vi "End Drag.vi"(8 "error in (no error)":errorcluster, 11 "FSM in":refnum<class "FSM.Node.lvclass">) -> (0 "error out":errorcluster, 3 "FSM out":refnum<class "FSM.Node.lvclass">)   [LabVIEW 2015, in "FSM.Node.lvclass"]
uses:
  FSM.Node.lvclass
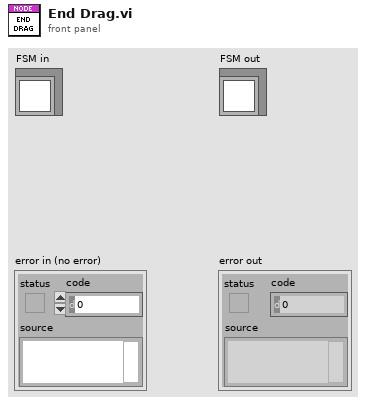
[diagram p1: front panel]
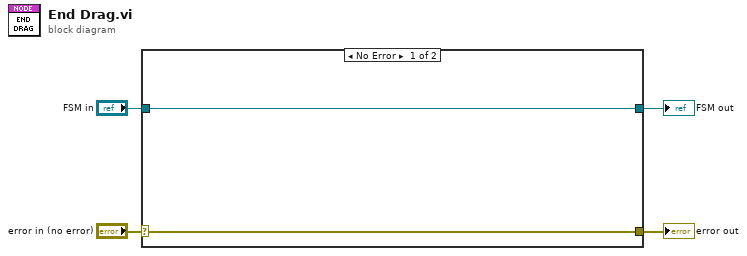
[diagram p0: block diagram]
diagram:
  n1 = case shown="No Error" "error in (no error)" {
    selector: "error in (no error)" -> [w6 w8]
    tunnel: [w6 w8] -> w3
    tunnel: [w5 w7] -> w1
    tunnel: "FSM in" -> [w5 w7]
    frame No Error {
    }
    frame Error {
    }
  }
  "error out" <- w3
  "FSM out" <- w1
